vi "Dwell Time.vi"(8 "error in (no error)":errorcluster, 10 "Dwell time (0.002 s)":dbl[unit]=0.002 format="%#_1g", 11 "VISA resource name":refnum<visa-resource-name>) -> (0 "error out":errorcluster, 3 "VISA resource name out":refnum<visa-resource-name>)   [LabVIEW 2015, in "SR400.lvlib"]
doc: "DT { x }\nThe DT command reads and sets the dwell time. If\nx is absent, the dwell time is returned. If x is\nincluded, the dwell time is set to x seconds where\n2E-3 <= x <= 6E1. If x = 0, the dwell is set to\nEXTERNAL. Only the most significant digit of x\nis used so \"DT 2E-3\" , \"DT .0022\" , \"DT 2.2E-3\"\nall set the dwell to 2 ms."
uses:
  SR400.lvlib
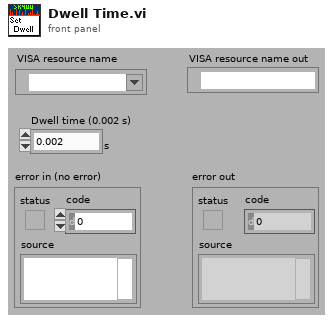
[diagram p1: front panel]
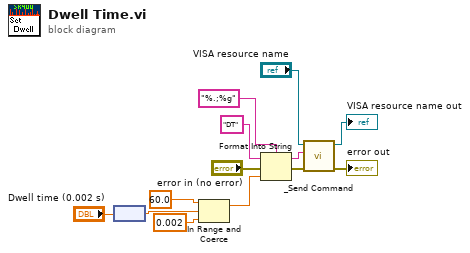
[diagram p0: block diagram]
diagram:
  n1 = node("Dwell time (0.002 s)") -> (w1:dbl)
  n2 = In Range and Coerce(upper limit=60.0, x=w1, lower limit=0.002) -> (coerced(x)=w5:dbl)  [unwired: 1 out]
  n3 = Format Into String(format string="%.;%g", initial string="DT" ("command"), error in="error in (no error)", w5) -> (resulting string=w9:string, error out=w8:errorcluster)
  n4 = call "_Send Command.vi"("error in (no error)"=w8, "Command"=w9, "VISA resource name"="VISA resource name") -> ("error out"=→"error out":errorcluster, "VISA resource name out"=→"VISA resource name out":refnum<visa-resource-name>)  [unwired: 1 in, 6 out]
